vi "Write Options.vi"(8 "error in (no error)":errorcluster, 10 "Options":T1[](array[typedef]), 11 "Beverage in":refnum<class "Beverage.lvclass">) -> (0 "error out":errorcluster, 3 "Beverage out":refnum<class "Beverage.lvclass">)   [LabVIEW 2023, in "Beverage.lvclass"]
doc: "Simple accessor method to write the <b>Options</b> of a Beverage."
uses:
  Beverage.lvclass
  TypeDefs/Options.ctl
  Beverage.lvclass/Beverage.ctl
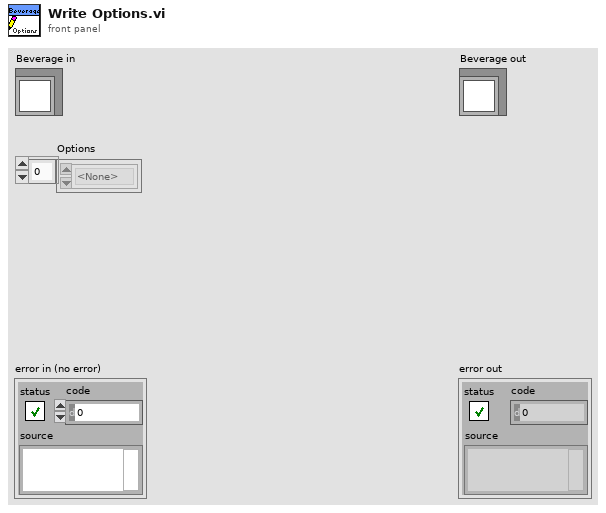
[diagram p1: front panel]
types:
  T1 = typedef "Beverage.lvclass/Options.ctl" = enum16{"<None>", "Milk", "Mocha", "Soy", "Whip"}
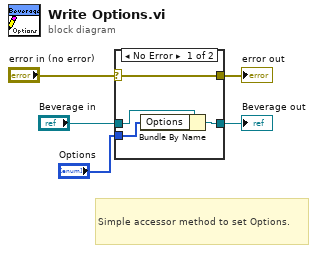
[diagram p0: block diagram]
diagram:
  # "Simple accessor method to set Options."
  n1 = case shown="No Error" "error in (no error)" {
    selector: "error in (no error)" -> [w9 w10]
    tunnel: [w9 w10] -> w4
    tunnel: [w7 w11] -> w2
    tunnel: "Beverage in" -> [w8 w11]
    tunnel: "Options" -> [w6 _]
    frame No Error {
      n2 = Bundle By Name(cluster=w8, "Options"=w6) -> (w7:refnum<class "Beverage.lvclass">)
    }
    frame Error {
    }
  }
  "error out" <- w4
  "Beverage out" <- w2
